vi "Image Fill.vi"(11 "image data in":T1) -> (3 "image data out":T1)   [LabVIEW 2018, in "Markdown.lvlib"]
doc: "Flood connector pane and icon 24-bit images to mask white (255, 255, 255)."
uses:
  Markdown.lvlib
  <vilib>/picture/picture.llb/imagedata.ctl
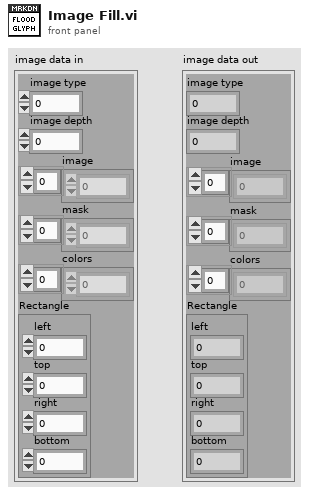
[diagram p1: front panel]
types:
  T1 = typedef "imagedata.ctl" = cluster{"image type":i32, "image depth":i32, "image":u8[], "mask":u8[], "colors":u32[], "Rectangle":cluster{"left":i16, "top":i16, "right":i16, "bottom":i16}}
  T2 = cluster{"left":i16, "top":i16, "right":i16, "bottom":i16}
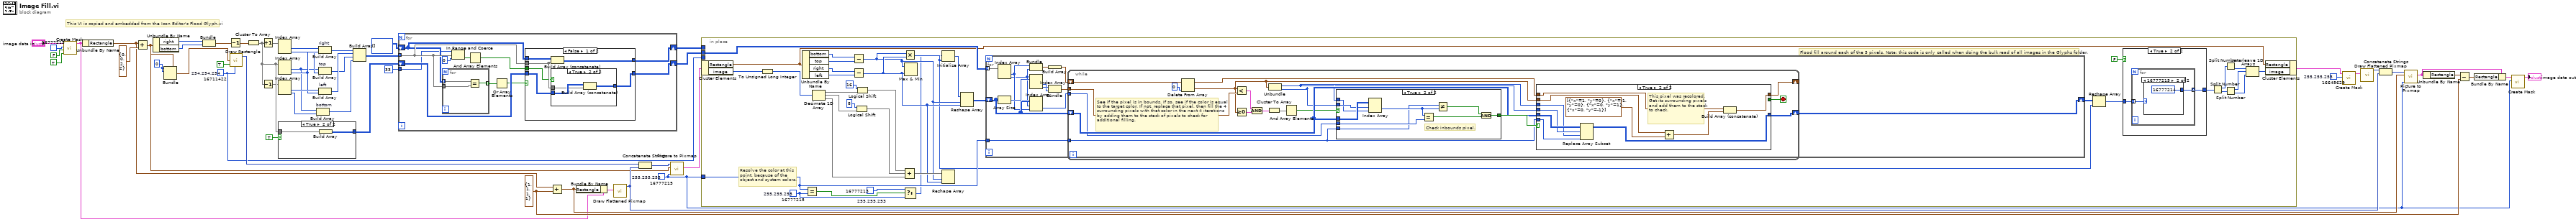
[diagram p0: block diagram]
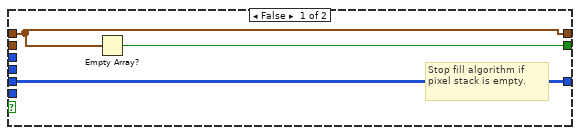
[diagram p6: hidden frame]
diagram:
  w18 = u32 16777215  # 255,255,255
  w2 = u32 16645629  # 255,255,253
  w45 = i16 0 ("left")
  w43 = u32 16711422  # 254.254.254
  w36 = T2 {"left"=1, "top"=1, "right"=1, "bottom"=1} ("y")
  # "This VI is copied and embedded from the Icon Editor's Flood Glyph.vi"
  n1 = call <vilib>:"Create Mask.vi"("Combine Masks? (F)"=TRUE, "1-Bit Mask Value (T)"=FALSE, "Mask Color (Black)"=u32 16777215, "image data"="image data in") -> ("image data"=w32:T1)  [unwired: 7 out]
  n2 = Unbundle By Name(w32) -> ("Rectangle"=w40:T2)
  n3 = Add(x=w40, y=T2 {"left"=0, "top"=0, "right"=2, "bottom"=2}) -> (x+y=w46:T2)
  n4 = Unbundle By Name(w46) -> ("right"=w51:i16, "bottom"=w52:i16)
  n5 = Bundle(cluster=w46, "left"=w45, "top"=w45) -> (w44:T2)  [unwired: 2 out]
  n6 = Bundle("right"=w51, "bottom"=w52) -> (w42:cluster{"right":i16, "bottom":i16})  [unwired: 1 out]
  n7 = Decrement(x=w42) -> (x-1=w39:cluster{"right":i16, "bottom":i16})
  n8 = call <vilib>:"Draw Rectangle.vi"("rect"=w44, "fill?(F)"=TRUE, "color(black)"=w43) -> ("new picture"=w53:picture)  [unwired: 6 in]
  n9 = Cluster To Array(cluster=w39) -> (array=w20:i16[])
  n10 = Increment(x=w20) -> (x+1=w14:i16[])
  n11 = Decrement(x=w20) -> (x-1=w13:i16[])
  n12 = Index Array(array=w14) -> (element #1=w12:i16, element #2=w9:i16)  [unwired: 2 in]
  n13 = Index Array(array=w20) -> (element #1=w8:i16, element #2=w10:i16)  [unwired: 2 in]
  n14 = Index Array(array=w13) -> (element #1=w11:i16, element #2=w7:i16)  [unwired: 2 in]
  n15 = case shown="True" TRUE ("Add Start Point?") {
    tunnel: [_ w56] -> w16
    tunnel: w20 -> [_ w55]
    frame False {
    }
    frame True {
      n16 = Build Array(w55) -> (w56:i16[][])
    }
  }
  n17 = Build Array "bottom"(w8, w7) -> (w3:i16[])
  n18 = Build Array "right"(w12, w10) -> (w6:i16[])
  n19 = Build Array "top"(w8, w9) -> (w4:i16[])
  n20 = Build Array "left"(w11, w10) -> (w5:i16[])
  n21 = Build Array(w6, w5, w4, w3) -> (w15:i16[][])
  n22 = for {
    tunnel: w15 -> [w62] mode=indexing
    shift-right: [w64] -> w21
    shift-left: w16 -> [w63]
    shift-right: [w59] -> w26
    shift-left: i32[][] [] ("Points In") -> [w58]
    tunnel: 33 ("#") -> [w57]
    n23 = for {
      tunnel: w58 -> [w82] mode=indexing
      tunnel: w62 -> [w81]
      tunnel: [w80] -> w61 mode=indexing
      n24 = Equal?(x=w82, y=w81) -> (x = y?=w80:bool)
    }
    n25 = In Range and Coerce(upper limit=w57, x=w62, lower limit=0) -> (In Range?=w66:bool[])  [unwired: 1 out]
    n26 = And Array Elements(Boolean array=w66) -> (logical AND=w65:bool)
    n27 = Or Array Elements(Boolean array=w61) -> (logical OR=w60:bool)
    n28 = case shown="False" w60 {
      tunnel: w65 -> [w68 _]
      tunnel: [w69 w79] -> w64
      tunnel: w63 -> [w73 w79]
      tunnel: w62 -> [w71 _]
      tunnel: w58 -> [w72 w78]
      tunnel: [w70 w78] -> w59
      frame False {
        n29 = Build Array (concatenate)(w72, w71) -> (w70:i32[][])
        n30 = case shown="True" w68 {
          tunnel: w73 -> [w74 w77]
          tunnel: w71 -> [_ w76]
          tunnel: [w74 w75] -> w69
          frame False {
          }
          frame True {
            n31 = Build Array (concatenate)(w77, w76) -> (w75:i16[][])
          }
        }
      }
      frame True {
      }
    }
  }
  n32 = Add(x=w40, y=w36) -> (x+y=w41:T2)
  n33 = Bundle By Name(cluster=w32, "Rectangle"=w41) -> (w50:T1)
  n34 = call <vilib>:"Draw Flattened Pixmap.vi"("image data"=w50) -> ("new picture"=w49:picture)  [unwired: 1 in, 7 out]
  n35 = Concatenate Strings(w53, w49) -> (w30:picture)
  n36 = call <vilib>:"Picture to Pixmap.vi"("Background Color"=w18, "rect"=w46, "picture"=w30) -> ("image data"=w24:T1)  [unwired: 1 in, 7 out]
  n37 = in-place {
    in-place-border: w21 -> [w118]
    in-place-border: w18 -> [w116]
    in-place-border: w43 -> [_]
    in-place-border: w26 -> [_]
    w100 = u32 16777213  # 255,255,253
    w101 = u32 16777215  # 255,255,255
    # "Flood fill around each of the 5 pixels. Note: this code is only called when doing the bulk read of all images in the Glyphs folder."
    # "Resolve the color at this\npoint, because of the\nobject and system colors."
    n38 = in-place-cluster #1(w24) -> ("Rectangle"=w113:T2, "image"=w115:u8[])
    n39 = To Unsigned Long Integer(number=w115) -> (unsigned 32bit integer=w109:u32[])
    n40 = Unbundle By Name(w113) -> ("bottom"=w95:i16, "top"=w94:i16, "right"=w93:i16, "left"=w92:i16)
    n41 = Equal?(x=w116, y=w101) -> (x = y?=w99:bool)
    n42 = Decimate 1D Array(w109) -> (w105:u32[], w111:u32[], w106:u32[])
    n43 = Subtract(x=w95, y=w94) -> (x-y=w97:i16)
    n44 = Subtract(x=w93, y=w92) -> (x-y=w98:i16)
    n45 = Logical Shift(y=i16 8, x=w111) -> (x << y=w112:u32[])
    n46 = Logical Shift(y=i16 16, x=w105) -> (x << y=w107:u32[])
    n47 = Multiply(x=w97, y=w98) -> (x*y=w96:i16)
    n48 = Select(t=w100, s=w99, f=w101) -> (s? t:f=w91:u32)
    n49 = Max & Min(x=w97, y=w98) -> ()  [unwired: 2 out]
    n50 = Compound Arithmetic op=ADD(w107, w112, w106) -> (w114:u32[])
    n51 = Initialize Array(w91, w96) -> (w84:u32[])
    n52 = Reshape Array(w114, w97, w98) -> ()  [unwired: 1 out]
    n53 = Reshape Array(w84, w97, w98) -> (w83:u32[][])
    n54 = for {
      tunnel: w116 -> [w126]
      shift-right: [w128] -> w85
      shift-left: w83 -> [w127]
      tunnel: w118 -> [w125] mode=indexing
      n55 = Index Array(array=w125) -> (element #1=w122:i16, element #2=w121:i16)  [unwired: 2 in]
      n56 = Array Size(array=w127) -> (size(s)=w129:i32[])
      n57 = Bundle("right"=w122, "right"=w121) -> (w123:cluster{"right":i16, "right":i16})  [unwired: 1 in]
      n58 = Index Array(array=w129) -> (element #1=w119:i32, element #2=w120:i32)  [unwired: 2 in]
      n59 = Index Array(array=w127, index (row)=w121, index (col)=w122) -> (element=w131:u32)
      n60 = Build Array(w123) -> (w130:cluster{"right":i16, "right":i16}[])
      n61 = Bundle(w120, w119) -> (w124:cluster{i32, i32})  [unwired: 1 in]
      n62 = while {
        shift-right: [w150] -> w128
        shift-left: w127 -> [w148]
        shift-right: [w147] -> _
        shift-left: w130 -> [w146]
        tunnel: w131 -> [w132]
        tunnel: w124 -> [w141]
        tunnel: w126 -> [w136]
        stop <- w137 stop-if-true
        # "See if the pixel is in bounds. If so, see if the color is equal to the target color. If not, replace that pixel, then fill the 4 surrounding pixels with that color in the next 4 iterations by adding them to the stack of pixels to check for additional filling."
        n63 = Delete From Array(array=w146, index=0) -> (deleted portion=w135:cluster{"right":i32, "right":i32}, array with subset deleted=w145:cluster{"right":i32, "right":i32}[])  [unwired: 1 in]
        n64 = Less?(x=w135, y=w141) -> (x < y?=w143:cluster{bool, bool})
        n65 = Greater Or Equal To 0?(x=w135) -> (x >= 0?=w142:cluster{"right":bool, "right":bool})
        n66 = Compound Arithmetic op=AND(w143, w142) -> (w140:cluster{bool, bool})
        n67 = Cluster To Array(cluster=w140) -> (array=w139:bool[])
        n68 = Unbundle(w135) -> ("right"=w134:i32, "right"=w133:i32)
        n69 = And Array Elements(Boolean array=w139) -> (logical AND=w138:bool)
        n70 = case shown="True" w138 {
          selector: w138 -> [w151 _]
          tunnel: w148 -> [_ w160]
          tunnel: [w151 w158] -> w149
          tunnel: w132 -> [_ w159]
          tunnel: w136 -> [_ w152]
          tunnel: w133 -> [_ w157]
          tunnel: w134 -> [_ w156]
          frame False {
            # "Pixel out of bounds."
          }
          frame True {
            # "Check inbounds pixel."
            n71 = Index Array(array=w160, index (row)=w157, index (col)=w156) -> (element=w155:u32)
            n72 = Equal?(x=w155, y=w159) -> (x = y?=w154:bool)
            n73 = Not Equal?(x=w152, y=w155) -> (x != y?=w153:bool)
            n74 = And(x=w153, y=w154) -> (x .and. y?=w158:bool)
          }
        }
        n75 = case shown="True" w149 {
          tunnel: w148 -> [w163 w173]
          tunnel: [w163 w172] -> w150
          tunnel: w136 -> [_ w171]
          tunnel: w134 -> [_ w167]
          tunnel: w133 -> [_ w168]
          tunnel: w135 -> [_ w166]
          tunnel: w145 -> [w162 w170]
          tunnel: [w162 w169] -> w147
          tunnel: [w161 _] -> w137
          frame False {
            # "Stop fill algorithm if pixel stack is empty."
            n76 = Empty Array?(array=w162) -> (empty?=w161:bool)
          }
          frame True {
            # "This pixel was recolored. Get its surrounding pixels and add them to the stack to check."
            n77 = Replace Array Subset(array=w173, new element=w171, index (row)=w168, index (col)=w167) -> (w172:u32[][])
            n78 = Add(x=w166, y=cluster{"x":i32, "y":i32}[] [{"x"=1, "y"=0}, {"x"=-1, "y"=0}, {"x"=0, "y"=1}, {"x"=0, "y"=-1}]) -> (x+y=w165:cluster{i32, i32}[])
            n79 = Build Array (concatenate)(w170, w165) -> (w169:cluster{"right":i32, "right":i32}[])
          }
        }
      }
    }
    n80 = Reshape Array(w85, w96) -> (w103:u32[])
    n81 = case shown="True" FALSE ("Swap Out White") {
      tunnel: [w174 w175] -> w102
      tunnel: w103 -> [w174 w176]
      frame False {
      }
      frame True {
        n82 = for {
          tunnel: w176 -> [w178] mode=indexing
          tunnel: [w177] -> w175 mode=indexing
          n83 = case shown="16777215" w178 {
            selector: w178 -> [w179 _]
            tunnel: [w179 u32 16777214 ("255,255,255")] -> w177
            frame Default {
            }
            frame 16777215 {
            }
          }
        }
      }
    }
    n84 = Split Number(x=w102) -> (hi(x)=w87:u16[], lo(x)=w86:u16[])
    n85 = Split Number(x=w87) -> (lo(x)=w88:u8[])  [unwired: 1 out]
    n86 = Split Number(x=w86) -> (hi(x)=w89:u8[], lo(x)=w90:u8[])
    n87 = Interleave 1D Arrays(w88, w89, w90) -> (w117:u8[])
    n88 = in-place-cluster #1("Rectangle"=w113, "image"=w117) -> (w22:T1)
  }
  n89 = call <vilib>:"Create Mask.vi"("Mask Color (Black)"=w2, "image data"=w22) -> ("image data"=w23:T1)  [unwired: 2 in, 7 out]
  n90 = call <vilib>:"Draw Flattened Pixmap.vi"("image data"=w23) -> ("new picture"=w38:picture)  [unwired: 1 in, 7 out]
  n91 = Concatenate Strings(w38, w49) -> (w47:picture)
  n92 = call <vilib>:"Picture to Pixmap.vi"("Background Color"=w18, "rect"=w41, "picture"=w47) -> ("image data"=w35:T1)  [unwired: 1 in, 7 out]
  n93 = Unbundle By Name(w35) -> ("Rectangle"=w37:T2)
  n94 = Subtract(x=w37, y=w36) -> (x-y=w34:T2)
  n95 = Bundle By Name(cluster=w35, "Rectangle"=w34) -> (w33:T1)
  n96 = call <vilib>:"Create Mask.vi"("Mask Color (Black)"=w18, "image data"=w33) -> ("image data"=→"image data out":T1)  [unwired: 2 in, 7 out]
